vi "624WPI_CameraRead MJPG for Dashboard.vi"(0 "Recording Name":string="Axis", 6 "Camera Settings":T2={"fps"=30, "compression"=30, "Image Size"=enum."320x240", "Config Shown"=FALSE}, 7 "Cam TCP Port":u16=1180, 8 "Rec Mode":u16(ring) items=["O", "*", "Open Playback Panel"], 9 "Camera IP":string, 10 "Camera Mode":u16(ring) items=["Camera Off", "USB Camera SW", "USB Camera HW", "IP Camera"], 11 "Refnum in":T1) -> (2 "Active":bool, 3 "Refnum out":T1, 4 "FPS":dbl, 5 "Bandwidth (Mbps)":dbl)   [LabVIEW 2017]
uses:
  <vilib>/Rock Robotics/WPI/Camera/WPI_CameraSettings Read MJPG.ctl
  <vilib>/Rock Robotics/WPI/Camera/WPI_CameraImageSize.ctl
  <vilib>/vision/Image Controls.llb/IMAQ Image.ctl
  <vilib>/Rock Robotics/WPI/Dashboard/WPI_DashboardLogging Global.vi
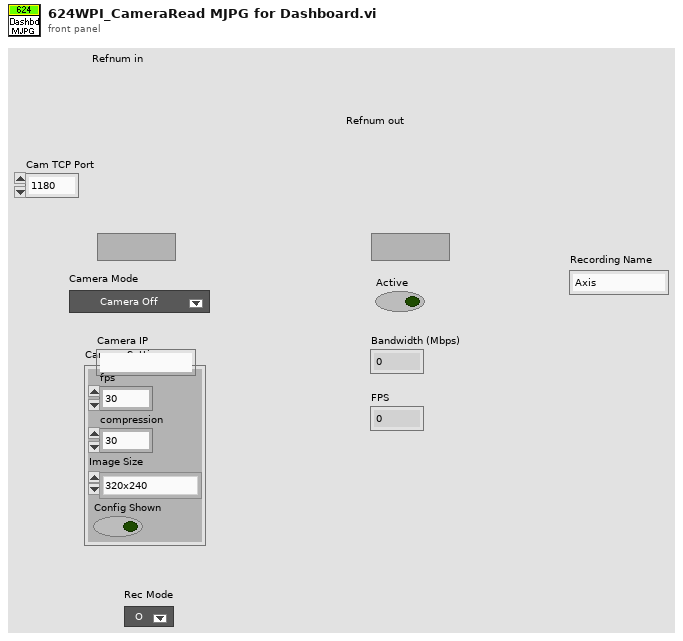
[diagram p1: front panel]
types:
  T1 = typedef "IMAQ Image.ctl" = refnum<image>
  T2 = typedef "WPI_CameraSettings Read MJPG.ctl" = cluster{"fps":i32, "compression":i32, "Image Size":T3, "Config Shown":bool}
  T3 = typedef "WPI_CameraImageSize.ctl" = enum16{"640x480", "320x240", "160x120", "Custom"}
  T4 = typedef "IMAQ AVI2 Refnum.ctl" = refnum<k20>
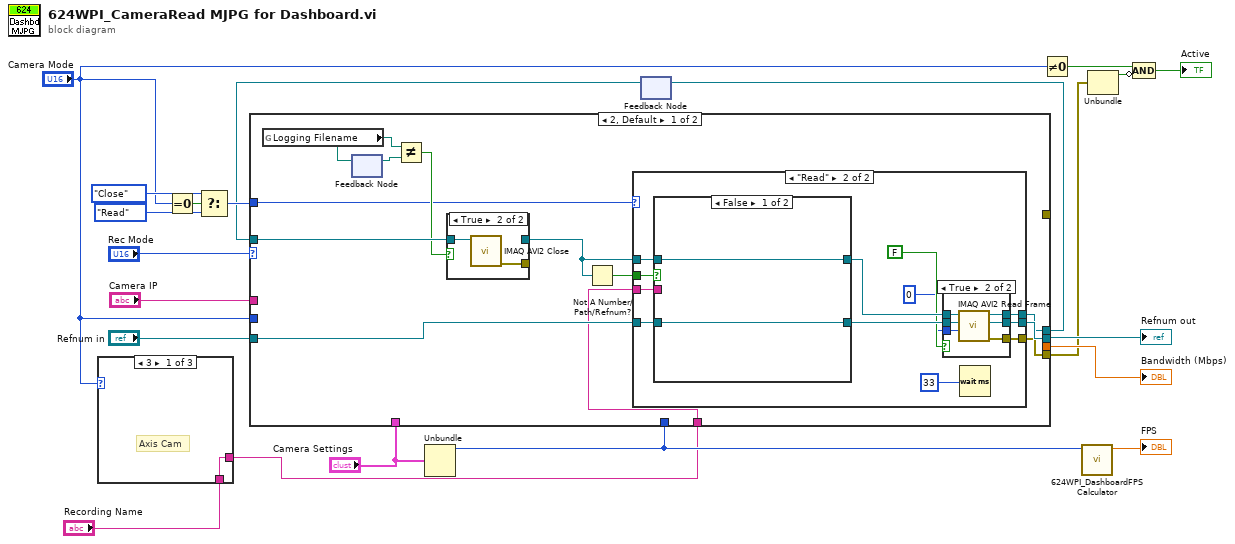
[diagram p0: block diagram]
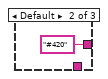
[diagram p2: hidden frame]
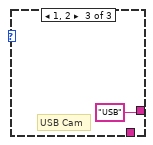
[diagram p3: hidden frame]
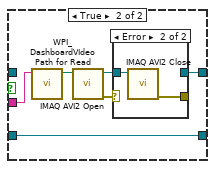
[diagram p6: hidden frame]
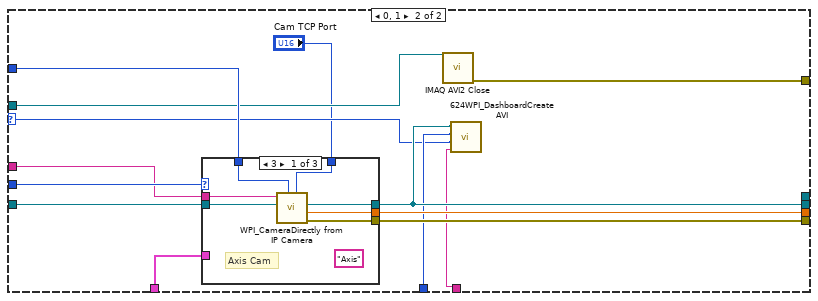
[diagram p9: hidden frame]
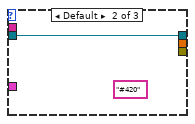
[diagram p10: hidden frame]
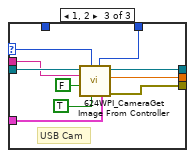
[diagram p11: hidden frame]
diagram:
  n1 = case shown="3" "Camera Mode" {
    tunnel: [w22 "#420" "USB"] -> w2
    tunnel: "Recording Name" -> [w22 _ _]
    frame 3 {
      # "Axis Cam"
    }
    frame Default {
    }
    frame 1, 2 {
      # "USB Cam"
    }
  }
  n2 = Equal To 0?(x="Camera Mode") -> (x = 0?=w7:bool)
  n3 = Select(t=enum16{"Read", "Reopen", "Close"}."Close" ("Operation"), s=w7, f=enum16{"Read", "Reopen", "Close"}."Read" ("Operation")) -> (s? t:f=w18:enum16{"Read", "Reopen", "Close"})
  n4 = Unbundle("Camera Settings") -> ("fps"=w5:i32)  [unwired: 3 out]
  n5 = feedback #1() -> (w10:T4)  [unwired: 1 in]
  n6 = case shown="2, Default" "Rec Mode" {
    selector: "Rec Mode" -> [_ w76]
    tunnel: "Camera Settings" -> [_ w86]
    tunnel: w18 -> [w26 w85]
    tunnel: [_ w84] -> w15
    tunnel: [w36 w78] -> w11
    tunnel: "Refnum in" -> [w34 w83]
    tunnel: "Camera IP" -> [_ w75]
    tunnel: w5 -> [_ w77]
    tunnel: w10 -> [w30 w81]
    tunnel: [w33 _] -> w9
    tunnel: [w32 w82] -> w8
    tunnel: [_ w80] -> _
    tunnel: "Camera Mode" -> [_ w79]
    tunnel: w2 -> [w25 w73]
    frame 2, Default {
      n7 = global read "WPI_DashboardLogging Global.vi" "Logging Filename"() -> (w29:path)
      n8 = feedback #2() -> (w28:path)  [unwired: 1 in]
      n9 = feedback-in #2(w29) -> ()
      n10 = Not Equal?(x=w29, y=w28) -> (x != y?=w27:bool)
      n11 = case shown="True" w27 {
        tunnel: [w70 _] -> w31
        tunnel: w30 -> [w70 w72]
        tunnel: [_ w71] -> _
        frame False {
        }
        frame True {
          n12 = call "IMAQ AVI2 Close"("AVI Refnum"=w72) -> ("error out"=w71:errorcluster)  [unwired: 10 in]
        }
      }
      n13 = Not A Number/Path/Refnum?(number/path/refnum=w31) -> (NaN/Path/Refnum?=w35:bool)
      n14 = case shown="\"Read\"" w26 {
        tunnel: [w37 w50] -> w36
        tunnel: w35 -> [_ w49]
        tunnel: w34 -> [w37 w46]
        tunnel: [w38 w45] -> w33
        tunnel: [_ w44] -> w32
        tunnel: w25 -> [_ w43]
        tunnel: w31 -> [w38 w42]
        frame "Close", Default {
        }
        frame "Read" {
          n15 = case shown="False" w49 {
            tunnel: [w60 w64] -> w48
            tunnel: w42 -> [w60 _]
            tunnel: [w59 w66] -> w47
            tunnel: w46 -> [w59 w66]
            tunnel: w43 -> [_ w62]
            frame False {
            }
            frame True {
              n16 = call <vilib>:"WPI_DashboardVIdeo Path for Read.vi"("Display Name"=w62) -> ("Video Path"=w61:path)  [unwired: 10 in]
              n17 = call "IMAQ AVI2 Open"("AVI File Path"=w61) -> ("error out"=w65:errorcluster, "AVI Refnum"=w63:T4)  [unwired: 9 in]
              n18 = case shown="Error" w65 {
                tunnel: [w67 _] -> w64
                tunnel: w63 -> [w67 w69]
                tunnel: [_ w68] -> _
                frame No Error {
                }
                frame Error {
                  n19 = call "IMAQ AVI2 Close"("AVI Refnum"=w69) -> ("error out"=w68:errorcluster)  [unwired: 10 in]
                }
              }
            }
          }
          n20 = case shown="True" FALSE {
            tunnel: [w51 w58] -> w50
            tunnel: w48 -> [w52 w57]
            tunnel: w47 -> [w51 w56]
            tunnel: [w52 w55] -> w45
            tunnel: [_ w54] -> w44
            tunnel: 0 -> [_ w53]
            frame False {
            }
            frame True {
              n21 = call "IMAQ AVI2 Read Frame"("Frame Number"=w53, "Image"=w56, "AVI Refnum"=w57) -> ("error out"=w54:errorcluster, "Image Out"=w58:T1, "AVI Refnum (duplicate)"=w55:T4)  [unwired: 6 in]
            }
          }
          n22 = Wait (ms)(milliseconds to wait=33) -> ()  [unwired: 1 out]
        }
      }
    }
    frame 0, 1 {
      n23 = case shown="3" w79 {
        selector: w79 -> [_ _ w97]
        tunnel: w86 -> [_ _ w99]
        tunnel: w85 -> [w88 _ _]
        tunnel: [w92 _ w98] -> w84
        tunnel: w83 -> [w90 w94 w104]
        tunnel: w75 -> [w89 _ w101]
        tunnel: [w93 _ w102] -> w82
        tunnel: [w91 w94 w103] -> w78
        tunnel: "Cam TCP Port" -> [w87 _ w96]
        frame 3 {
          (unwired) "Axis"
          # "Axis Cam"
          n24 = call <vilib>:"WPI_CameraDirectly from IP Camera.vi"("port"=w87, "Operation"=w88, "Image"=w90, "address"=w89) -> ("error out"=w93:errorcluster, "Bandwidth (Mbps)"=w92:dbl, "Image Out"=w91:T1)  [unwired: 5 in]
        }
        frame Default {
          (unwired) "#420"
        }
        frame 1, 2 {
          # "USB Cam"
          n25 = call "624WPI_CameraGet Image From Controller.vi"("Camera Settings"=w99, "port"=w96, "USB"=TRUE, "Camera Mode"=w97, "Close?"=FALSE, "Controller Address"=w101, "Image"=w104) -> ("error out"=w102:errorcluster, "Bandwidth (Mbps)"=w98:dbl, "Image Out"=w103:T1)  [unwired: 2 in]
        }
      }
      n26 = call "IMAQ AVI2 Close"("AVI Refnum"=w81) -> ("error out"=w80:errorcluster)  [unwired: 10 in]
      n27 = call "624WPI_DashboardCreate AVI.vi"("Camera IP"=w73, "Recording"=w76, "frames per seconds"=w77, "Image"=w78) -> ()  [unwired: 8 in]
    }
  }
  "Bandwidth (Mbps)" <- w15
  "Refnum out" <- w11
  n28 = feedback-in #1(w9) -> ()
  n29 = Not Equal To 0?(x="Camera Mode") -> (x != 0?=w6:bool)
  n30 = call "624WPI_DashboardFPS Calculator.vi"("Average Count"=w5) -> ("fps"=→"FPS":dbl)  [unwired: 10 in]
  n31 = Unbundle(w8) -> ("status"=w19:bool)  [unwired: 2 out]
  n32 = Compound Arithmetic op=AND(w6, invert w19) -> (→"Active":bool)
